vi "Write ID.vi"(8 "error in (no error)":errorcluster, 10 "ID":string, 11 "Generic Update Data Message in":refnum<class "Generic Update Data Message.lvclass">) -> (0 "error out":errorcluster, 3 "Generic Update Data Message out":refnum<class "Generic Update Data Message.lvclass">)   [LabVIEW 2014, in "DAQ Device.lvlib" / "Generic Update Data Message.lvclass"]
uses:
  Generic Update Data Message.lvclass
  Generic Update Data Message.lvclass/Generic Update Data Message.ctl
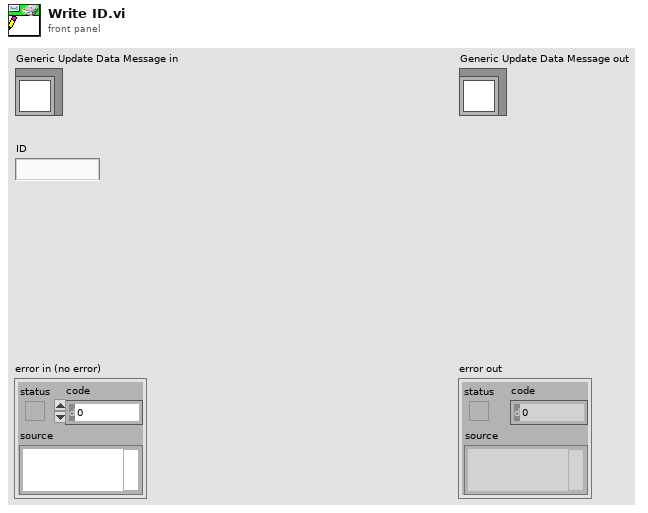
[diagram p1: front panel]
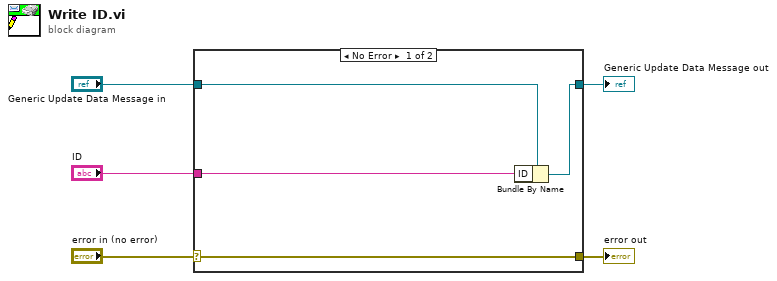
[diagram p0: block diagram]
diagram:
  n1 = case shown="No Error" "error in (no error)" {
    selector: "error in (no error)" -> [w9 w10]
    tunnel: [w9 w10] -> w4
    tunnel: [w7 w11] -> w2
    tunnel: "Generic Update Data Message in" -> [w8 w11]
    tunnel: "ID" -> [w6 _]
    frame No Error {
      n2 = Bundle By Name(cluster=w8, "ID"=w6) -> (w7:refnum<class "Generic Update Data Message.lvclass">)
    }
    frame Error {
    }
  }
  "error out" <- w4
  "Generic Update Data Message out" <- w2
